vi "BOOL.vi"() -> ()   [LabVIEW 2020]
panel:
  out "OR 2":bool
  out "NOT":bool
  out "XOR":bool
  out "OR":bool
  out "AND":bool
  in  "Boolean 2":bool
  in  "Boolean":bool
  # "BOOLEANOS"
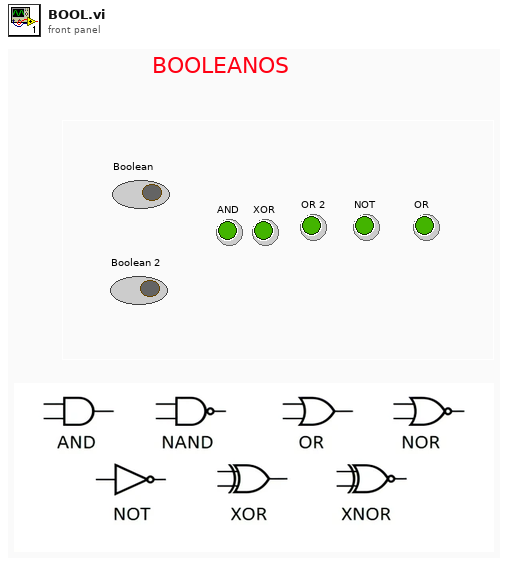
[diagram p1: front panel]
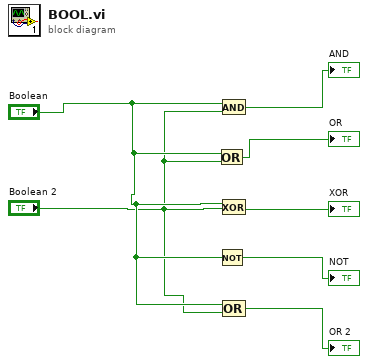
[diagram p0: block diagram]
diagram:
  n1 = Or(x="Boolean", y="Boolean 2") -> (x .or. y?=→"OR":bool)
  n2 = Not(x="Boolean") -> (.not. x?=→"NOT":bool)
  n3 = And(x="Boolean", y="Boolean 2") -> (x .and. y?=→"AND":bool)
  n4 = Exclusive Or(1:"Boolean 2", 2:"Boolean") -> (0:→"XOR":bool)
  n5 = Compound Arithmetic op=OR("Boolean", "Boolean 2") -> (→"OR 2":bool)
